vi "NewVIObjectOwnerByUID.vi"(5 "vi object class":refnum<vi>, 6 "location":T1, 7 "style":i32, 8 "error in (no error)":errorcluster, 10 "owner":cluster{"owner?":bool, "ownerUID":i32}, 11 "targetVI":refnum<vi>) -> (0 "error out":errorcluster, 1 "UID":i32, 2 "object refnum":refnum<vi>, 3 "dup targetVI":refnum<vi>)   [LabVIEW 2013]
uses:
  <vilib>/Utility/miscctls.llb/LVPointTypeDef.ctl
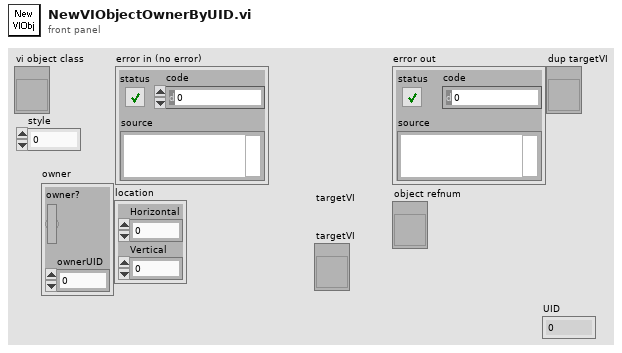
[diagram p1: front panel]
types:
  T1 = typedef "LVPointTypeDef.ctl" = cluster{"Horizontal":i16, "Vertical":i16}
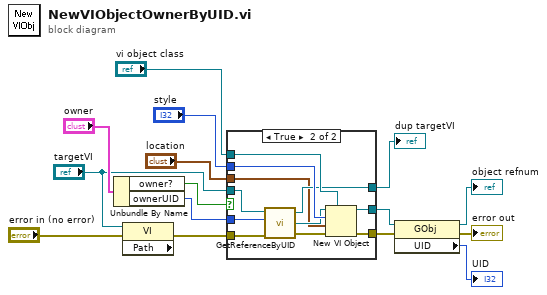
[diagram p0: block diagram]
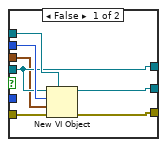
[diagram p2: hidden frame]
diagram:
  n1 = Unbundle By Name("owner") -> ("owner?"=w15:bool, "ownerUID"=w14:i32)
  n2 = property class="VI" props=["Path"](reference="targetVI", error in="error in (no error)") -> (error out=w1:errorcluster)  [unwired: 2 out]
  n3 = case shown="True" w15 {
    tunnel: w1 -> [w21 w32]
    tunnel: "targetVI" -> [w17 w33]
    tunnel: w14 -> [_ w31]
    tunnel: [w22 w24] -> w5
    tunnel: [w19 w29] -> w8
    tunnel: "vi object class" -> [w18 w28]
    tunnel: "style" -> [w20 w27]
    tunnel: [w17 w25] -> w10
    tunnel: "location" -> [w16 w23]
    frame False {
      n4 = New VI Object(vi object class=w18, owner refnum=w17, style=w20, position/next to=w16, 8:w21) -> (object refnum=w19:refnum<vi>, 0:w22:errorcluster)  [unwired: 3 in]
    }
    frame True {
      n5 = call "GetReferenceByUID.vi"("error in (no error)"=w32, "UID"=w31, "targetVI"=w33) -> ("error out"=w30:errorcluster, "refNum"=w26:refnum<vi>, "dup targetVI"=w25:refnum<vi>)  [unwired: 1 in]
      n6 = New VI Object(vi object class=w28, owner refnum=w26, style=w27, position/next to=w23, 8:w30) -> (object refnum=w29:refnum<vi>, 0:w24:errorcluster)  [unwired: 3 in]
    }
  }
  "dup targetVI" <- w10
  n7 = property class="GObj"(reference=w8, error in=w5) -> (reference out=→"object refnum":refnum<vi>, error out=→"error out":errorcluster, "UID"=→"UID":i32)
